vi "Read Waveform.vi"(8 "error in (no error)":errorcluster, 9 "Type":waveform(dbl), 10 "Tag":string, 11 "Var Bus in":refnum<class "Omni_Bus.lvclass">) -> (0 "error out":errorcluster, 2 "Waveform":waveform(dbl), 3 "Var Bus out":refnum<class "Omni_Bus.lvclass">)   [LabVIEW 2021, in "Omni_Bus.lvclass"]
uses:
  Omni_Bus.lvclass
  <vilib>/TSA/Abstract Data Classes/Abs_Types/Waveform/Abs_Waveform.lvclass
  Omni_Bus.lvclass/Omni_Bus.ctl
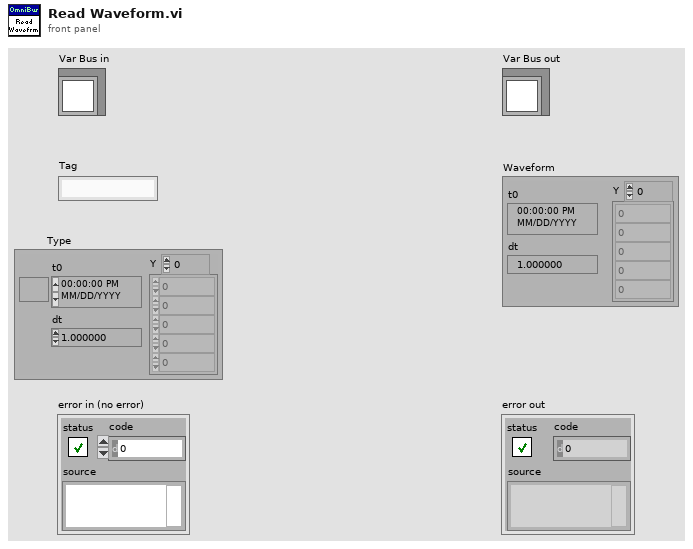
[diagram p1: front panel]
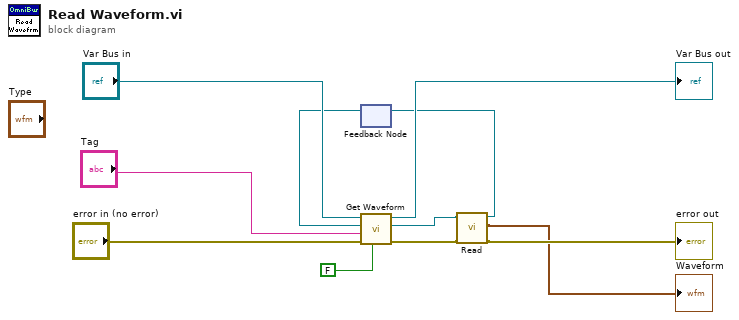
[diagram p0: block diagram]
diagram:
  n1 = feedback #1() -> (w7:refnum<class "Abs_Waveform.lvclass">)  [unwired: 1 in]
  n2 = call-dynamic "Get Waveform.vi"("Write?"=FALSE, "error in (no error)"="error in (no error)", "Tag"="Tag", "Value Type"=w7, "Var Bus in"="Var Bus in") -> ("error out"=w6:errorcluster, "Value Out"=w5:refnum<class "Abs_Waveform.lvclass">, "Var Bus out"=→"Var Bus out":refnum<class "Omni_Bus.lvclass">)  [unwired: 4 in]
  n3 = call-dynamic "Read.vi"("error in (no error)"=w6, "Abs_Waveform in"=w5) -> ("error out"=→"error out":errorcluster, "Waveform"=→"Waveform":waveform(dbl), "Abs_Waveform out"=w3:refnum<class "Abs_Waveform.lvclass">)  [unwired: 7 in]
  n4 = feedback-in #1(w3) -> ()
